vi "PositionControl_y_4mode.vi"() -> ()   [LabVIEW 2014]
uses:
  <vilib>/rvi/FXPMathLib/FxpSinAndCos/subVIs/nifxpmath_SinAndCos_SimConfig.ctl
  <vilib>/rvi/Emulation/niFpgaGetClockAttributes.vi
  <vilib>/rvi/Emulation/niFpgaSctlEmulationGetInTimedLoop.vi
  <vilib>/rvi/Emulation/niFpgaEmulationReportErrorSimple.vi
  <vilib>/rvi/eio/common/nirviEmuTemplateMethod_errors.vi
  <vilib>/rvi/Emulation/niFpgaProcessEmulError.vi
  <vilib>/rvi/Emulation/niFpgaCriticalErrorInLSC.vi
  <vilib>/rvi/FXPMathLib/FxpSinAndCos/simVIs/DllFxpSinAndCosTemp_sub.vi
  <vilib>/rvi/interface/RandomDataEmulation/nirviRandomDataMultiElementFPGAFIFO.vi
  <instcachedir>/0/nirviRandomDataMultiElementFPGAFIFO_AD0CFC12EF974623A9C2E4184BC062B2.lvgen/nirviRandomDataMultiElementFPGAFIFO_AD0CFC12EF974623A9C2E4184BC062B2_020.vi
  <vilib>/rvi/interface/RandomDataEmulation/niFpgaRandomDataHandleErrors.vi
  <vilib>/eio/EIONode/EIONode.xnode
  <vilib>/rvi/FXPMathLib/FxpMul/XNode/nifxpmath_Multiplier.xnode
  <vilib>/rvi/FXPMathLib/FxpSinAndCos/XNode/nifxpmath_SinAndCos.xnode
  <vilib>/rvi/Analysis/measure/butterworth/XNode/niFpgaButterworthFilter.xnode
  <vilib>/rvi/FXPMathLib/FxpSub/XNode/nifxpmath_Sub.xnode
  <vilib>/rvi/FXPMathLib/FxpAdd/XNode/nifxpmath_Add.xnode
  <vilib>/rvi/DataTransferAndStorage/Container/XNode/niFpgaContainer.xnode
  <vilib>/rvi/interface/RandomDataEmulation/nirviRandomDataFpgaMultiElementTemplate.vi
  <vilib>/rvi/FXPMathLib/sim/FxpSim.dll
panel:
  in  "Frequency_start (Hz)":fxp<+/-,20,5>
  in  "Target time (s)":fxp<+/-,24,9>
  in  "Frequency_end (Hz)":fxp<+/-,23,8>
  out "Chirp_signal":fxp<+/-,36,11>
  in  "Chirp ampitude (mm)":fxp<+/-,20,11>
  out "omega (M_avg)":fxp<+/-,64,35>
  out "D_d (M_avg)":fxp<+/-,64,32>
  in  "D_d_M_avg_Tc (uSec)":u32
  out "omega (M)":fxp<+/-,64,30>
  out "D_d (M)":fxp<+/-,64,27>
  in  "D_d_M_Tc (uSec)":u32 format="%#_6f"
  out "D_d (T)":fxp<+/-,46,10>
  out "omega(T)":fxp<+/-,20,9>
  in  "Velocity Estimation":i16(ring) items=["M_avg method", "M method", "T method"]
  out "Dr_ramp":fxp<+/-,64,30>
  out "Dr_slope":fxp<+/-,33,17>
  in  "Dr_time":fxp<+/-,16,11>
  out "Dr_sin":fxp<+/-,28,11>
  out "Dr_sin_d":fxp<+/-,64,16>
  out "Dr_sin_dd":fxp<+/-,64,25>
  out "Sin omega":fxp<+/-,41,8>
  in  "Sin offset":fxp<+/-,27,10>
  in  "Sin magnitude":fxp<+/-,11,8>
  in  "Sin wave frequency (Hz)":fxp<+/-,21,5>
  out "Time now (s)":fxp<+,52,14>
  out "Dr":fxp<+/-,64,31>
  in  "Dr_end":fxp<+/-,16,11>
  in  "Command type":i16(ring) items=["Step", "Ramp", "Sine", "Chirp"]
  out "D_i":fxp<+/-,34,18>
  in  "D_tolorence":fxp<+/-,14,3>
  in  "Ki":fxp<+/-,20,6>
  out "D_error":fxp<+/-,24,11>
  in  "Direction":bool
  out "Fmr_PD":fxp<+/-,64,31>
  in  "Kd":fxp<+/-,20,8>
  in  "Kp":fxp<+/-,20,12>
  in  "scaled coefficients_D_dd":i32[](array[numeric])=[780119100, 146811362]
  out "D_dd":fxp<+/-,36,29>
  in  "Ini coe.":bool
  out "va":fxp<+/-,38,8>
  out "vb":fxp<+/-,38,8>
  in  "stop motor":bool
  out "vq_F":fxp<+/-,20,5> format="%.57g"
  out "vd_F":fxp<+/-,20,5>
  out "D_d (mm/s)":fxp<+/-,32,12>
  out "mt":u32
  out "omega (rad/s)":fxp<+/-,32,18>
  in  "mt0":u32
  out "D(mm)":fxp<+/-,22,8>
  out "rad(NrTheta)":fxp<+/-,33,18>
  out "Encoder Position":i32
  in  "Encoder Reset":bool
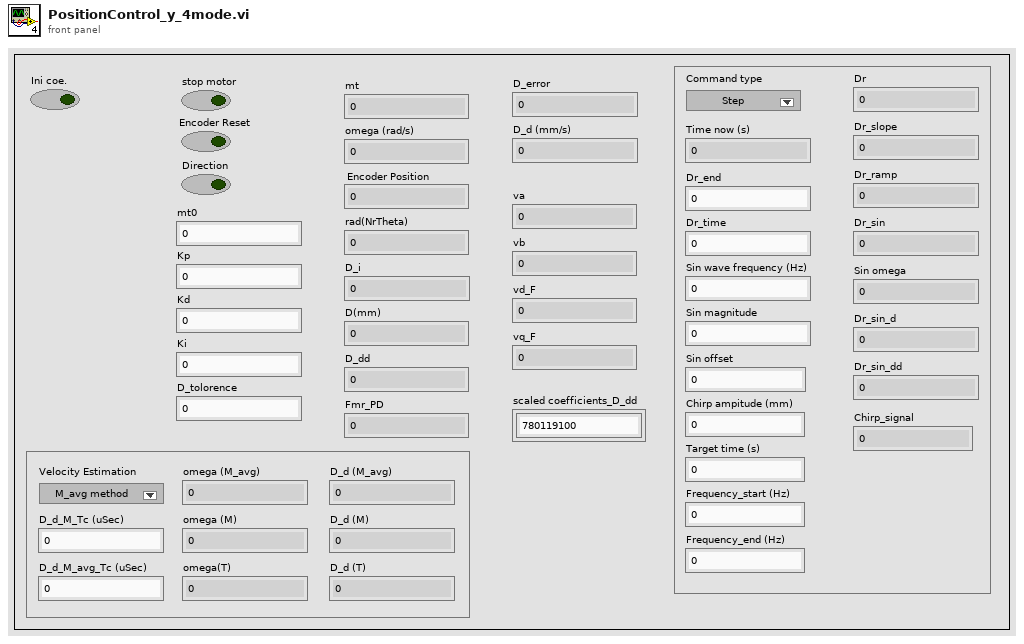
[diagram p1: front panel]
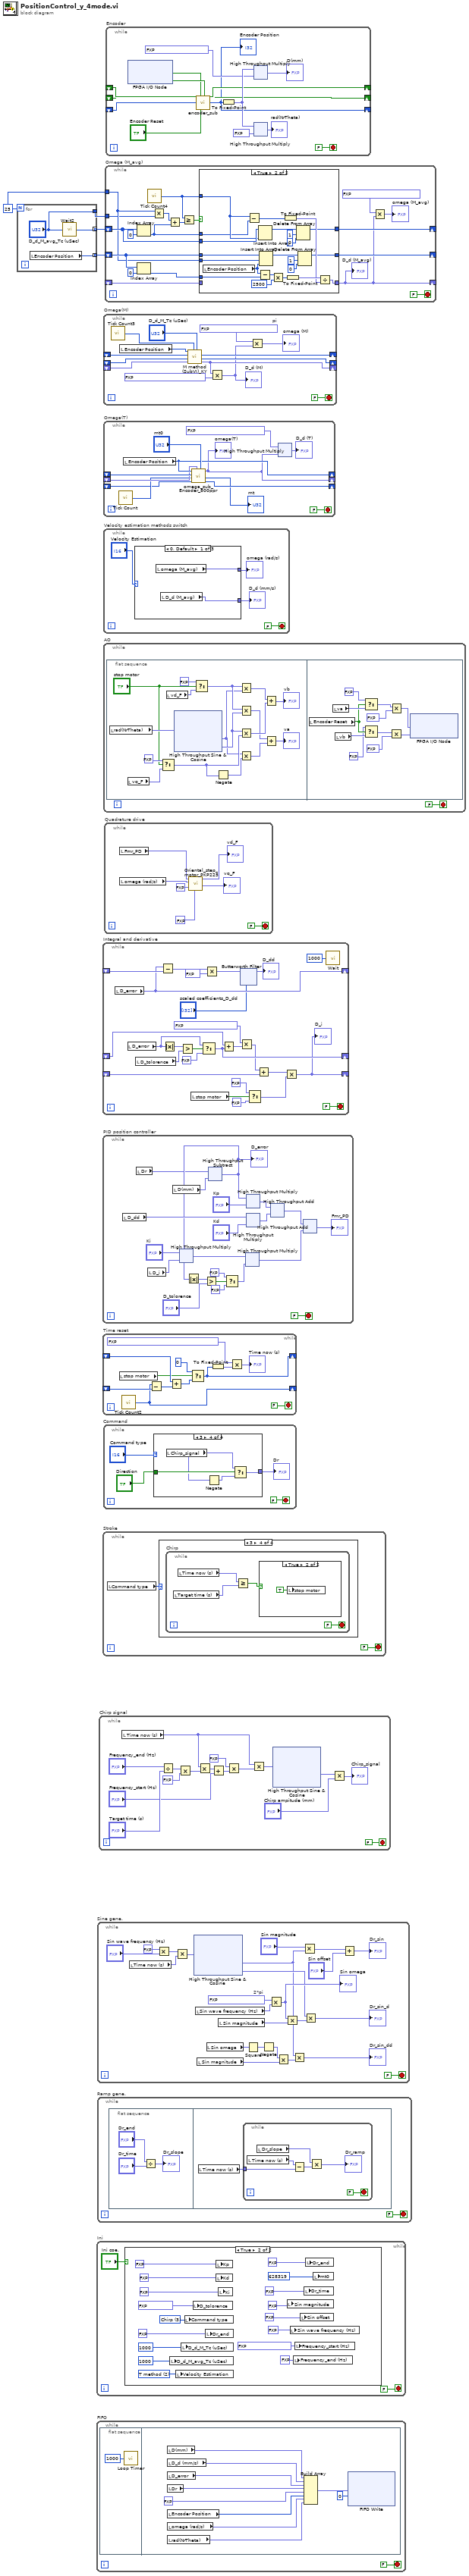
[diagram p0: block diagram]
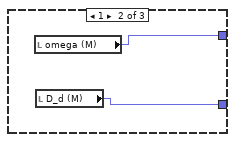
[diagram p3: hidden frame]
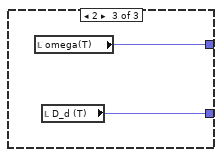
[diagram p4: hidden frame]
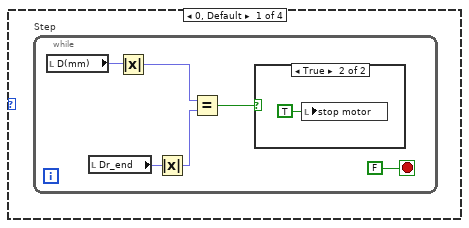
[diagram p5: hidden frame]
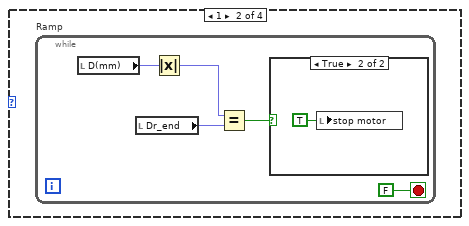
[diagram p7: hidden frame]
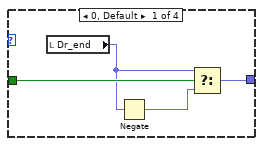
[diagram p11: hidden frame]
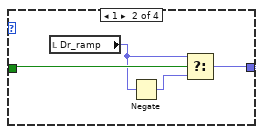
[diagram p12: hidden frame]
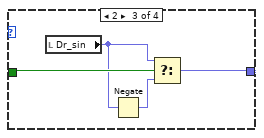
[diagram p13: hidden frame]
diagram:
  w4 = 25
  n1 = for {
    N: w4 -> [_]
    tunnel: ["D_d_M_avg_Tc (uSec)"] -> w1
    tunnel: [w6] -> w3 mode=indexing
    tunnel: [w5] -> w2 mode=indexing
    n2 = local read "Encoder Position"() -> (w5:i32)
    n3 = call "Wait2"("Count(uSec)"="D_d_M_avg_Tc (uSec)") -> ("Tick Count(uSec)"=w6:u32)
  }
  n4 = while "Ini" {
    stop <- FALSE stop-if-true
    n5 = case shown="True" "Ini coe." {
      frame False {
      }
      frame True {
        w10 = i16 3 items=["Step", "Ramp", "Sine", "Chirp"] ("Command type")
        w13 = i16 2 items=["M_avg method", "M method", "T method"] ("Velocity Estimation")
        n6 = local write "D_d_M_avg_Tc (uSec)"(u32 1000 ("D_d_M_avg_Tc (uSec)")) -> ()
        n7 = local write "Velocity Estimation"(w13) -> ()
        n8 = local write "D_d_M_Tc (uSec)"(u32 1000 ("D_d_M_Tc (uSec)")) -> ()
        n9 = local write "Command type"(w10) -> ()
        n10 = local write "D_tolorence"(fxp<+/-,14,3> 0.009765625 ("D_tolorence")) -> ()
        n11 = local write "Dr_end"(fxp<+/-,16,11> 20.0 ("Dr_end")) -> ()
        n12 = local write "Kp"(fxp<+/-,20,12> 15.0 ("Kp")) -> ()
        n13 = local write "Kd"(fxp<+/-,20,8> 0.0 ("Kd")) -> ()
        n14 = local write "Ki"(fxp<+/-,20,6> 0.0 ("D_i")) -> ()
        n15 = local write "Sin magnitude"(fxp<+/-,11,8> 20.0 ("Sin magnitude")) -> ()
        n16 = local write "Sin wave frequency (Hz)"(fxp<+/-,21,5> 0.5 ("Sin wave frequency (Hz)")) -> ()
        n17 = local write "Frequency_end (Hz)"(fxp<+/-,23,8> 10.0 ("Frequency_end (Hz)")) -> ()
        n18 = local write "Frequency_start (Hz)"(fxp<+/-,20,5> 0.100006103515625 ("Frequency_start (Hz)")) -> ()
        n19 = local write "Sin offset"(fxp<+/-,27,10> 0.0 ("Sin offset")) -> ()
        n20 = local write "Dr_time"(fxp<+/-,16,11> 30.0 ("Dr_time")) -> ()
        n21 = local write "Dr_end"(fxp<+/-,11,7> 20.0 ("Fmr")) -> ()
        n22 = local write "mt0"(u32 628319 ("mt0")) -> ()
      }
    }
  }
  n23 = while "FIFO" {
    stop <- FALSE stop-if-true
    n24 = flat-sequence {
      frame #0 {
        n25 = call "Loop Timer"("Count(uSec)"=u32 1000) -> ()  [unwired: 1 out]
      }
      frame #1 {
        n26 = local read "D(mm)"() -> (w36:fxp<+/-,22,8>)
        n27 = local read "D_d (mm/s)"() -> (w35:fxp<+/-,32,12>)
        n28 = local read "D_error"() -> (w34:fxp<+/-,24,11>)
        n29 = local read "Dr"() -> (w33:fxp<+/-,64,31>)
        n30 = local read "Encoder Position"() -> (w32:i32)
        n31 = local read "omega (rad/s)"() -> (w31:fxp<+/-,32,18>)
        n32 = local read "rad(NrTheta)"() -> (w30:fxp<+/-,33,18>)
        n33 = Build Array(w36, w35, w34, w33, fxp<+/-,64,32> 0.0 ("element"), w32, w31, w30) -> (w37:fxp<+/-,64,32>[])
        n34 = xnode ("FIFO Write")("Element"=w37, "Timeout"=0) -> ()  [unwired: 1 in, 2 out]
      }
    }
  }
  n35 = while "Sine gene." {
    stop <- FALSE stop-if-true
    w56 = fxp<+,20,3> 6.2831878662109375  # 2*pi
    n36 = local read "Time now (s)"() -> (w59:fxp<+,52,14>)
    n37 = Multiply(x=fxp<+,1,2> 2.0, y="Sin wave frequency (Hz)") -> (x*y=w60:fxp<+/-,21,6>)
    n38 = Multiply(x=w60, y=w59) -> (x*y=w40:fxp<+/-,64,20>)
    n39 = xnode "High Throughput Sine & Cosine"("x (pi)"=w40) -> ("sin(x)"=w44:fxp<+/-,16,2>, "cos(x)"=w51:fxp<+/-,16,2>)
    n40 = local read "Sin wave frequency (Hz)"() -> (w55:fxp<+/-,21,5>)
    n41 = local read "Sin magnitude"() -> (w46:fxp<+/-,11,8>)
    n42 = local read "Sin omega"() -> (w47:fxp<+/-,41,8>)
    n43 = local read "Sin magnitude"() -> (w50:fxp<+/-,11,8>)
    n44 = Square(x=w47) -> (x^2=w48:fxp<+,64,14>)
    n45 = Negate(x=w48) -> (-x=w45:fxp<+/-,64,15>)
    n46 = Multiply(x=w56, y=w55) -> (x*y=w52:fxp<+/-,41,8>)
    "Sin omega" <- w52
    n47 = Multiply(x=w45, y=w46) -> (x*y=w49:fxp<+/-,64,23>)
    n48 = Multiply(x=w52, y=w50) -> (x*y=w57:fxp<+/-,51,15>)
    n49 = Multiply(x=w44, y=w49) -> (x*y=→"Dr_sin_dd":fxp<+/-,64,25>)
    n50 = Multiply(x="Sin magnitude", y=w44) -> (x*y=w58:fxp<+/-,27,10>)
    n51 = Multiply(x=w51, y=w57) -> (x*y=→"Dr_sin_d":fxp<+/-,64,16>)
    n52 = Add(x=w58, y="Sin offset") -> (x+y=→"Dr_sin":fxp<+/-,28,11>)
  }
  n53 = while "Ramp gene." {
    stop <- FALSE stop-if-true
    n54 = flat-sequence {
      frame #0 {
        n55 = Divide(x="Dr_end", y="Dr_time") -> (x/y=→"Dr_slope":fxp<+/-,33,17>)
      }
      frame #1 {
        n56 = local read "Time now (s)"() -> (w97:fxp<+,52,14>)
        n57 = while {
          tunnel: w97 -> [w103]
          stop <- FALSE stop-if-true
          n58 = local read "Time now (s)"() -> (w100:fxp<+,52,14>)
          n59 = local read "Dr_slope"() -> (w101:fxp<+/-,33,17>)
          n60 = Subtract(x=w100, y=w103) -> (x-y=w102:fxp<+/-,53,15>)
          n61 = Multiply(x=w101, y=w102) -> (x*y=→"Dr_ramp":fxp<+/-,64,30>)
        }
      }
    }
  }
  n62 = while "Chirp signal" {
    stop <- FALSE stop-if-true
    n63 = local read "Time now (s)"() -> (w110:fxp<+,52,14>)
    n64 = Divide(x="Frequency_end (Hz)", y="Target time (s)") -> (x/y=w113:fxp<+/-,24,9>)
    n65 = Multiply(x=w113, y=fxp<+/-,24,9> 0.5) -> (x*y=w111:fxp<+/-,23,10>)
    n66 = Multiply(x=w110, y=w111) -> (x*y=w109:fxp<+/-,26,11>)
    n67 = Add(x=w109, y="Frequency_start (Hz)") -> (x+y=w107:fxp<+/-,20,5>)
    n68 = Multiply(x=fxp<+/-,3,3> 2.0, y=w107) -> (x*y=w105:fxp<+/-,25,10>)
    n69 = Multiply(x=w110, y=w105) -> (x*y=w116:fxp<+/-,33,18>)
    n70 = xnode "High Throughput Sine & Cosine"("x (pi)"=w116) -> ("sin(x)"=w119:fxp<+/-,16,2>)  [unwired: 1 out]
    n71 = Multiply(x=w119, y="Chirp ampitude (mm)") -> (x*y=→"Chirp_signal":fxp<+/-,36,11>)
  }
  n72 = while "Integral and derivative" {
    shift-right: [w170] -> _
    shift-left: _ -> [w174]
    shift-right: [w160] -> _
    shift-left: _ -> [w161]
    shift-right: [w150] -> _
    shift-left: _ -> [w154]
    stop <- FALSE stop-if-true
    n73 = local read "D_error"() -> (w170:fxp<+/-,24,11>)
    n74 = local read "D_error"() -> (w162:fxp<+/-,24,11>)
    n75 = local read "D_tolorence"() -> (w165:fxp<+/-,14,3>)
    n76 = Subtract(x=w170, y=w174) -> (x-y=w173:fxp<+/-,25,12>)
    n77 = Absolute Value(x=w162) -> (abs(x)=w166:fxp<+,24,11>)
    n78 = Greater?(x=w166, y=w165) -> (0:w164:bool)
    n79 = local read "stop motor"() -> (w157:bool)
    n80 = Select(t=w162, s=w164, f=fxp<+,24,11> 0.0) -> (s? t:f=w160:fxp<+/-,25,12>)
    n81 = Multiply(x=w173, y=fxp<+/-,33,13> 1000.0) -> (x*y=w171:fxp<+/-,57,24>)
    n82 = Add(x=w161, y=w160) -> (x+y=w159:fxp<+/-,26,13>)
    n83 = Multiply(x=fxp<+/-,30,12> 0.000499725341796875, y=w159) -> (x*y=w153:fxp<+/-,55,24>)
    n84 = xnode "Butterworth Filter"("input data"=w171, "scaled coefficients"="scaled coefficients_D_dd") -> ("output data"=→"D_dd":fxp<+/-,36,28>)  [unwired: 1 in]
    n85 = Select(t=fxp<+,1,1> 0.0, s=w157, f=fxp<+,1,1> 1.0) -> (s? t:f=w151:fxp<+,1,1>)
    n86 = Add(x=w153, y=w154) -> (x+y=w152:fxp<+/-,32,16>)
    n87 = Multiply(x=w152, y=w151) -> (x*y=w150:fxp<+/-,32,16>)
    "D_i" <- w150
    n88 = call "Wait"("Count(uSec)"=u32 1000) -> ()  [unwired: 1 out]
  }
  n89 = while "PID position controller" {
    stop <- FALSE stop-if-true
    n90 = local read "D_dd"() -> (w200:fxp<+/-,36,29>)
    n91 = local read "Dr"() -> (w184:fxp<+/-,64,31>)
    n92 = local read "D_i"() -> (w195:fxp<+/-,34,18>)
    n93 = local read "D(mm)"() -> (w204:fxp<+/-,22,8>)
    n94 = xnode ("High Throughput Multiply")("x"="Ki", "y"=w195) -> ("x*y"=w189:fxp<+/-,54,24>)
    n95 = xnode "High Throughput Subtract"("x"=w184, "y"=w204) -> ("x-y"=w193:fxp<+/-,64,32>)
    "D_error" <- w193
    n96 = Absolute Value(x=w193) -> (abs(x)=w194:fxp<+,64,32>)
    n97 = Greater?(x=w194, y="D_tolorence") -> (0:w192:bool)
    n98 = Select(t=fxp<+,10,2> 1.0, s=w192, f=fxp<+,10,2> 0.0) -> (s? t:f=w188:fxp<+,10,2>)
    n99 = xnode ("High Throughput Multiply")("x"=w189, "y"=w188) -> ("x*y"=w185:fxp<+/-,64,26>)
    n100 = xnode ("High Throughput Multiply")("x"=w193, "y"="Kp") -> ("x*y"=w202:fxp<+/-,64,44>)
    n101 = xnode ("High Throughput Multiply")("x"=w200, "y"="Kd") -> ("x*y"=w201:fxp<+/-,56,37>)
    n102 = xnode ("High Throughput Add")("x"=w202, "y"=w201) -> ("x+y"=w186:fxp<+/-,64,45>)
    n103 = xnode ("High Throughput Add")("x"=w186, "y"=w185) -> ("x+y"=→"Fmr_PD":fxp<+/-,64,46>)
  }
  n104 = while "Time reset" {
    shift-right: [w208] -> _
    shift-left: _ -> [w215]
    shift-right: [w210] -> _
    shift-left: _ -> [w211]
    stop <- FALSE stop-if-true
    n105 = local read "stop motor"() -> (w213:bool)
    n106 = call "Tick Count2"() -> ("Tick Count(uSec)"=w210:u32)
    n107 = Subtract(x=w210, y=w211) -> (x-y=w216:u32)
    n108 = Add(x=w215, y=w216) -> (x+y=w214:u32)
    n109 = Select(t=u32 0, s=w213, f=w214) -> (s? t:f=w208:u32)
    n110 = To Fixed-Point(number=w208) -> (fixed-point=w207:fxp<+,32,32>)  [unwired: 1 in]
    n111 = Multiply(x=fxp<+,20,-18> 1.0000003385357559e-06, y=w207) -> (x*y=→"Time now (s)":fxp<+,52,14>)
  }
  n112 = while "Stroke" {
    stop <- FALSE stop-if-true
    n113 = local read "Command type"() -> (w218:i16)
    n114 = case shown="3" w218 {
      frame 0, Default {
        n115 = while "Step" {
          stop <- FALSE stop-if-true
          n116 = local read "D(mm)"() -> (w222:fxp<+/-,22,8>)
          n117 = local read "Dr_end"() -> (w224:fxp<+/-,16,11>)
          n118 = Absolute Value(x=w222) -> (abs(x)=w219:fxp<+,22,8>)
          n119 = Absolute Value(x=w224) -> (abs(x)=w223:fxp<+,16,11>)
          n120 = Equal?(x=w219, y=w223) -> (x = y?=w221:bool)
          n121 = case shown="True" w221 {
            frame False {
            }
            frame True {
              n122 = local write "stop motor"(TRUE ("stop motor")) -> ()
            }
          }
        }
      }
      frame 1 {
        n123 = while "Ramp" {
          stop <- FALSE stop-if-true
          n124 = local read "D(mm)"() -> (w230:fxp<+/-,22,8>)
          n125 = local read "Dr_end"() -> (w229:fxp<+/-,16,11>)
          n126 = Absolute Value(x=w230) -> (abs(x)=w226:fxp<+,22,8>)
          n127 = Equal?(x=w226, y=w229) -> (x = y?=w228:bool)
          n128 = case shown="True" w228 {
            frame False {
            }
            frame True {
              n129 = local write "stop motor"(TRUE ("stop motor")) -> ()
            }
          }
        }
      }
      frame 2 {
      }
      frame 3 {
        n130 = while "Chirp" {
          stop <- FALSE stop-if-true
          n131 = local read "Target time (s)"() -> (w234:fxp<+/-,24,9>)
          n132 = local read "Time now (s)"() -> (w235:fxp<+,52,14>)
          n133 = Greater Or Equal?(x=w235, y=w234) -> (x >= y?=w233:bool)
          n134 = case shown="True" w233 {
            frame False {
            }
            frame True {
              n135 = local write "stop motor"(TRUE ("stop motor")) -> ()
            }
          }
        }
      }
    }
  }
  n136 = while "Command" {
    stop <- FALSE stop-if-true
    n137 = case shown="3" "Command type" {
      tunnel: [w241 w245 w249 w253] -> w239
      tunnel: "Direction" -> [w244 w248 w252 w256]
      frame 0, Default {
        n138 = local read "Dr_end"() -> (w243:fxp<+/-,16,11>)
        n139 = Negate(x=w243) -> (-x=w242:fxp<+/-,17,12>)
        n140 = Select(t=w243, s=w244, f=w242) -> (s? t:f=w241:fxp<+/-,17,12>)
      }
      frame 1 {
        n141 = local read "Dr_ramp"() -> (w246:fxp<+/-,64,30>)
        n142 = Negate(x=w246) -> (-x=w247:fxp<+/-,64,31>)
        n143 = Select(t=w246, s=w248, f=w247) -> (s? t:f=w245:fxp<+/-,64,31>)
      }
      frame 2 {
        n144 = local read "Dr_sin"() -> (w250:fxp<+/-,28,11>)
        n145 = Negate(x=w250) -> (-x=w251:fxp<+/-,27,10>)
        n146 = Select(t=w250, s=w252, f=w251) -> (s? t:f=w249:fxp<+/-,28,11>)
      }
      frame 3 {
        n147 = local read "Chirp_signal"() -> (w254:fxp<+/-,36,11>)
        n148 = Negate(x=w254) -> (-x=w255:fxp<+/-,37,12>)
        n149 = Select(t=w254, s=w256, f=w255) -> (s? t:f=w253:fxp<+/-,37,12>)
      }
    }
    "Dr" <- w239
  }
  n150 = while "Omega(M)" {
    shift-right: [w268] -> _
    shift-left: _ -> [w269]
    shift-right: [w264] -> _
    shift-left: _ -> [w265]
    shift-right: [w262] -> _
    shift-left: _ -> [w263]
    stop <- FALSE stop-if-true
    w259 = fxp<+/-,27,3> 3.1415926218032837  # pi
    n151 = call "Tick Count3"() -> ("Tick Count(mSec)"=w267:u32)
    n152 = local read "Encoder Position"() -> (w270:i32)
    n153 = call "M method (SubVI)_KY.vi"("Tc (mSec)"="D_d_M_Tc (uSec)", "Tick Count (mSec)"=w267, "Encoder velocity_pre (pulse/s)"=w263, "Shift Register in 2"=w265, "Shift Register in 1"=w269, "Encoder pulses"=w270) -> ("Encoder velocity (pulse/s)"=w262:fxp<+/-,64,32>, "Shift Register out 2"=w264:i32, "Shift Register out 1"=w268:u32)  [unwired: 3 in]
    n154 = Multiply(x=w262, y=fxp<+/-,20,-5> 0.002499997615814209) -> (x*y=w260:fxp<+/-,64,27>)
    "D_d (M)" <- w260
    n155 = Multiply(x=w259, y=w260) -> (x*y=→"omega (M)":fxp<+/-,64,30>)
  }
  n156 = while "Omega(T)" {
    shift-right: [w280] -> _
    shift-left: _ -> [w281]
    shift-right: [w273] -> _
    shift-left: _ -> [w279]
    shift-right: [w276] -> _
    shift-left: _ -> [w277]
    stop <- FALSE stop-if-true
    n157 = call "Tick Count"() -> ("Tick Count(Ticks)"=w278:u32)
    n158 = local read "Encoder Position"() -> (w280:i32)
    n159 = call "omega_sub_Encoder_800ppr.vi"("mt0"="mt0", "omega_pre"=w279, "ticks_m_pre"=w277, "ticks"=w278, "count_pre"=w281, "count"=w280) -> ("ticks_m"=w276:u32, "mt"=→"mt":u32, "omega"=w273:fxp<+/-,20,9>)  [unwired: 3 in]
    "omega(T)" <- w273
    n160 = xnode ("High Throughput Multiply")("x"=fxp<+/-,26,1> 0.3183099031448364, "y"=w273) -> ("x*y"=→"D_d (T)":fxp<+/-,46,10>)
  }
  n161 = while "Velocity estimation methods switch" {
    stop <- FALSE stop-if-true
    n162 = case shown="0, Default" "Velocity Estimation" {
      tunnel: [w288 w290 w292] -> w285
      tunnel: [w287 w289 w291] -> w284
      frame 0, Default {
        n163 = local read "omega (M_avg)"() -> (w288:fxp<+/-,64,35>)
        n164 = local read "D_d (M_avg)"() -> (w287:fxp<+/-,64,32>)
      }
      frame 1 {
        n165 = local read "omega (M)"() -> (w290:fxp<+/-,64,30>)
        n166 = local read "D_d (M)"() -> (w289:fxp<+/-,64,27>)
      }
      frame 2 {
        n167 = local read "omega(T)"() -> (w292:fxp<+/-,20,9>)
        n168 = local read "D_d (T)"() -> (w291:fxp<+/-,46,10>)
      }
    }
    "D_d (mm/s)" <- w284
    "omega (rad/s)" <- w285
  }
  n169 = while "AO" {
    stop <- FALSE stop-if-true
    n170 = flat-sequence {
      frame #0 {
        n171 = local read "rad(NrTheta)"() -> (w309:fxp<+/-,33,18>)
        n172 = local read "vq_F"() -> (w307:fxp<+/-,20,5>)
        n173 = Select(t=fxp<+,20,5> 0.0, s="stop motor", f=w307) -> (s? t:f=w304:fxp<+/-,21,6>)
        n174 = local read "vd_F"() -> (w308:fxp<+/-,20,5>)
        n175 = xnode "High Throughput Sine & Cosine"("x (pi)"=w309) -> ("sin(x)"=w300:fxp<+/-,17,2>, "cos(x)"=w302:fxp<+/-,17,2>)
        n176 = Select(t=fxp<+,20,5> 0.0, s="stop motor", f=w308) -> (s? t:f=w301:fxp<+/-,21,6>)
        n177 = Negate(x=w304) -> (-x=w303:fxp<+/-,21,6>)
        n178 = Multiply(x=w301, y=w300) -> (x*y=w299:fxp<+/-,37,7>)
        n179 = Multiply(x=w301, y=w302) -> (x*y=w297:fxp<+/-,37,7>)
        n180 = Multiply(x=w302, y=w304) -> (x*y=w298:fxp<+/-,37,7>)
        n181 = Multiply(x=w300, y=w303) -> (x*y=w296:fxp<+/-,37,7>)
        n182 = Add(x=w299, y=w298) -> (x+y=→"vb":fxp<+/-,38,8>)
        n183 = Add(x=w297, y=w296) -> (x+y=→"va":fxp<+/-,38,8>)
      }
      frame #1 {
        n184 = local read "Encoder Reset"() -> (w343:bool)
        n185 = local read "va"() -> (w345:fxp<+/-,38,8>)
        n186 = local read "vb"() -> (w344:fxp<+/-,38,8>)
        n187 = Select(t=fxp<+/-,20,5> 5.0 ("y"), s=w343, f=w345) -> (s? t:f=w346:fxp<+/-,38,8>)
        n188 = Select(t=fxp<+/-,20,5> 0.0 ("y"), s=w343, f=w344) -> (s? t:f=w347:fxp<+/-,38,8>)
        n189 = Multiply(x=w347, y=fxp<+/-,20,5> -0.5) -> (x*y=w351:fxp<+/-,57,12>)
        n190 = Multiply(x=w346, y=fxp<+/-,20,5> -0.5) -> (x*y=w350:fxp<+/-,57,12>)
        n191 = xnode "FPGA I/O Node"("Mod8/AO2"=w350, "Mod8/AO3"=w351) -> ()  [unwired: 2 in, 2 out]
      }
    }
  }
  n192 = while "Quadrature drive" {
    stop <- FALSE stop-if-true
    n193 = local read "Fmr_PD"() -> (w352:fxp<+/-,64,31>)
    n194 = local read "omega (rad/s)"() -> (w354:fxp<+/-,32,18>)
    n195 = call "Oriental_step_motor_PKP225.vi"("F_Threshold"=fxp<+,12,12> 10.0, "dFmr"=fxp<+/-,25,15> 0.0, "omega"=w354, "Fmr"=w352) -> ("vq_F"=→"vq_F":fxp<+/-,20,5>, "vd_F"=→"vd_F":fxp<+/-,20,5>)  [unwired: 6 in]
  }
  n196 = while "Omega (M_avg)" {
    tunnel: w4 -> [w370]
    shift-right: [w363] -> _
    shift-left: w3 -> [w374]
    shift-right: [w362] -> _
    shift-left: _ -> [w365]
    shift-right: [w364] -> _
    shift-left: w2 -> [w373]
    tunnel: w1 -> [w367]
    stop <- FALSE stop-if-true
    n197 = Index Array(array=w374, index=0) -> (element=w368:u32)
    n198 = Index Array(array=w373, index=0) -> (element=w369:i32)
    n199 = call "Tick Count4"() -> ("Tick Count(uSec)"=w371:u32)
    n200 = Multiply(x=w370, y=w367) -> (x*y=w375:u32)
    n201 = Add(x=w375, y=w368) -> (x+y=w372:u32)
    n202 = Greater Or Equal?(x=w371, y=w372) -> (x >= y?=w366:bool)
    n203 = case shown="True" w366 {
      tunnel: w374 -> [w380 w397]
      tunnel: w373 -> [w379 w396]
      tunnel: w371 -> [_ w389]
      tunnel: w370 -> [_ w395]
      tunnel: w369 -> [_ w393]
      tunnel: w368 -> [_ w388]
      tunnel: w365 -> [w378 _]
      tunnel: [w379 w383] -> w364
      tunnel: [w380 w382] -> w363
      tunnel: [w378 w381] -> w362
      frame False {
      }
      frame True {
        n204 = local read "Encoder Position"() -> (w394:i32)
        n205 = Subtract(x=w389, y=w388) -> (x-y=w386:u32)
        n206 = Insert Into Array(array=w397, new element=w389) -> (w398:u32[])  [unwired: 1 in]
        n207 = Subtract(x=w394, y=w393) -> (x-y=w392:i32)
        n208 = Insert Into Array(array=w396, index=w395, new element=w394) -> (w399:i32[])
        n209 = Multiply(x=w392, y=2500) -> (x*y=w390:i32)
        n210 = To Fixed-Point(number=w386) -> (fixed-point=w384:fxp<+,32,32>)  [unwired: 1 in]
        n211 = To Fixed-Point(number=w390) -> (fixed-point=w385:fxp<+/-,32,32>)  [unwired: 1 in]
        n212 = Delete From Array(array=w398, length=1, index=0) -> (array with subset deleted=w382:u32[])  [unwired: 1 out]
        n213 = Delete From Array(array=w399, length=1, index=0) -> (array with subset deleted=w383:i32[])  [unwired: 1 out]
        n214 = Divide(x=w385, y=w384) -> (x/y=w381:fxp<+/-,64,32>)
      }
    }
    "D_d (M_avg)" <- w362
    n215 = Multiply(x=fxp<+/-,27,3> 3.1415926218032837, y=w362) -> (x*y=→"omega (M_avg)":fxp<+/-,64,35>)
  }
  n216 = while "Encoder" {
    shift-right: [w409] -> _
    shift-left: _ -> [w411]
    shift-right: [w408] -> _
    shift-left: _ -> [w410]
    shift-right: [w406] -> _
    shift-left: _ -> [w407]
    stop <- FALSE stop-if-true
    n217 = xnode "FPGA I/O Node"() -> ("Mod4/DI0"=w416:bool, "Mod4/DI1"=w417:bool)  [unwired: 2 in, 2 out]
    n218 = call "encoder_sub.vi"("A_pre"=w411, "B_pre"=w410, "Encoder Position_pre"=w407, "A input"=w416, "Encoder Position Reset"="Encoder Reset", "B input"=w417) -> ("A"=w409:bool, "B"=w408:bool, "Encoder Position (Counts)"=w406:i32)  [unwired: 19 in]
    "Encoder Position" <- w406
    n219 = To Fixed-Point(number=w406) -> (fixed-point=w414:fxp<+/-,32,32>)  [unwired: 1 in]
    n220 = xnode ("High Throughput Multiply")("x"=w414, "y"=fxp<+/-,24,0> 0.003055572509765625) -> ("x*y"=→"D(mm)":fxp<+/-,56,32>)
    n221 = xnode ("High Throughput Multiply")("x"=w414, "y"=fxp<+/-,24,0> 0.125) -> ("x*y"=→"rad(NrTheta)":fxp<+/-,56,32>)
  }
